vi "Set 2D Ramp Rates_manual_ramp_brasse.vi"(0 "Y-Axis Communications Config":T1={"GPIB address"=22, "GPIB bus"=0, "connection ID"=refnum, "IP"="192.168.2.200", "Active Comm Interface"=0, "Serial Port"="", "Programmer Type"=0} {"Programmer Type" items=["Model 430", "Model 420"]; "Active Comm Interface" items=["TCP/IP (Model 430 Only)", "RS232", "IEEE488"]}, 1 "Y-Axis Field (kG)":dbl format="%.3f", 3 "Next Y-Axis Field (kG)":dbl format="%.3f", 4 "Z-Axis Communications Config":T1={"GPIB address"=22, "GPIB bus"=0, "connection ID"=refnum, "IP"="192.168.2.200", "Active Comm Interface"=0, "Serial Port"="", "Programmer Type"=0} {"Programmer Type" items=["Model 430", "Model 420"]; "Active Comm Interface" items=["TCP/IP (Model 430 Only)", "RS232", "IEEE488"]}, 5 "Z-Axis Field (kG)":dbl format="%.3f", 6 "User defined Ramp Rate (T/min)":bool, 7 "Next Z-Axis Field (kG)":dbl format="%.3f", 8 "Max Ramp Rate - Y Axis (A/s)":dbl format="%.3f", 9 "Max Ramp Rate - Z Axis (A/s)":dbl format="%.3f", 10 "User defined Ramp Rate - Z Axis (kG/s)":dbl format="%.3f", 11 "error in":T2, 12 "User defined Ramp Rate Y-Axis (kG/s)":dbl format="%.3f") -> (15 "Y-Axis Ramp Rate (T/min)":dbl format="%.3f", 17 "Z-Axis Ramp Rate (T/min)":dbl format="%.3f", 18 "error out":T2)   [LabVIEW 2009]
panel:
  in  "Z-Axis Communications Config 4":T1={"GPIB address"=22, "GPIB bus"=0, "connection ID"=refnum, "IP"="192.168.2.200", "Active Comm Interface"=0, "Serial Port"="", "Programmer Type"=0} {"Programmer Type" items=["Model 430", "Model 420"]; "Active Comm Interface" items=["TCP/IP (Model 430 Only)", "RS232", "IEEE488"]}
  in  "Z-Axis Communications Config 3":T1={"GPIB address"=22, "GPIB bus"=0, "connection ID"=refnum, "IP"="192.168.2.200", "Active Comm Interface"=0, "Serial Port"="", "Programmer Type"=0} {"Programmer Type" items=["Model 430", "Model 420"]; "Active Comm Interface" items=["TCP/IP (Model 430 Only)", "RS232", "IEEE488"]}
  in  "Z-Axis Communications Config 2":T1={"GPIB address"=22, "GPIB bus"=0, "connection ID"=refnum, "IP"="192.168.2.200", "Active Comm Interface"=0, "Serial Port"="", "Programmer Type"=0} {"Programmer Type" items=["Model 430", "Model 420"]; "Active Comm Interface" items=["TCP/IP (Model 430 Only)", "RS232", "IEEE488"]}
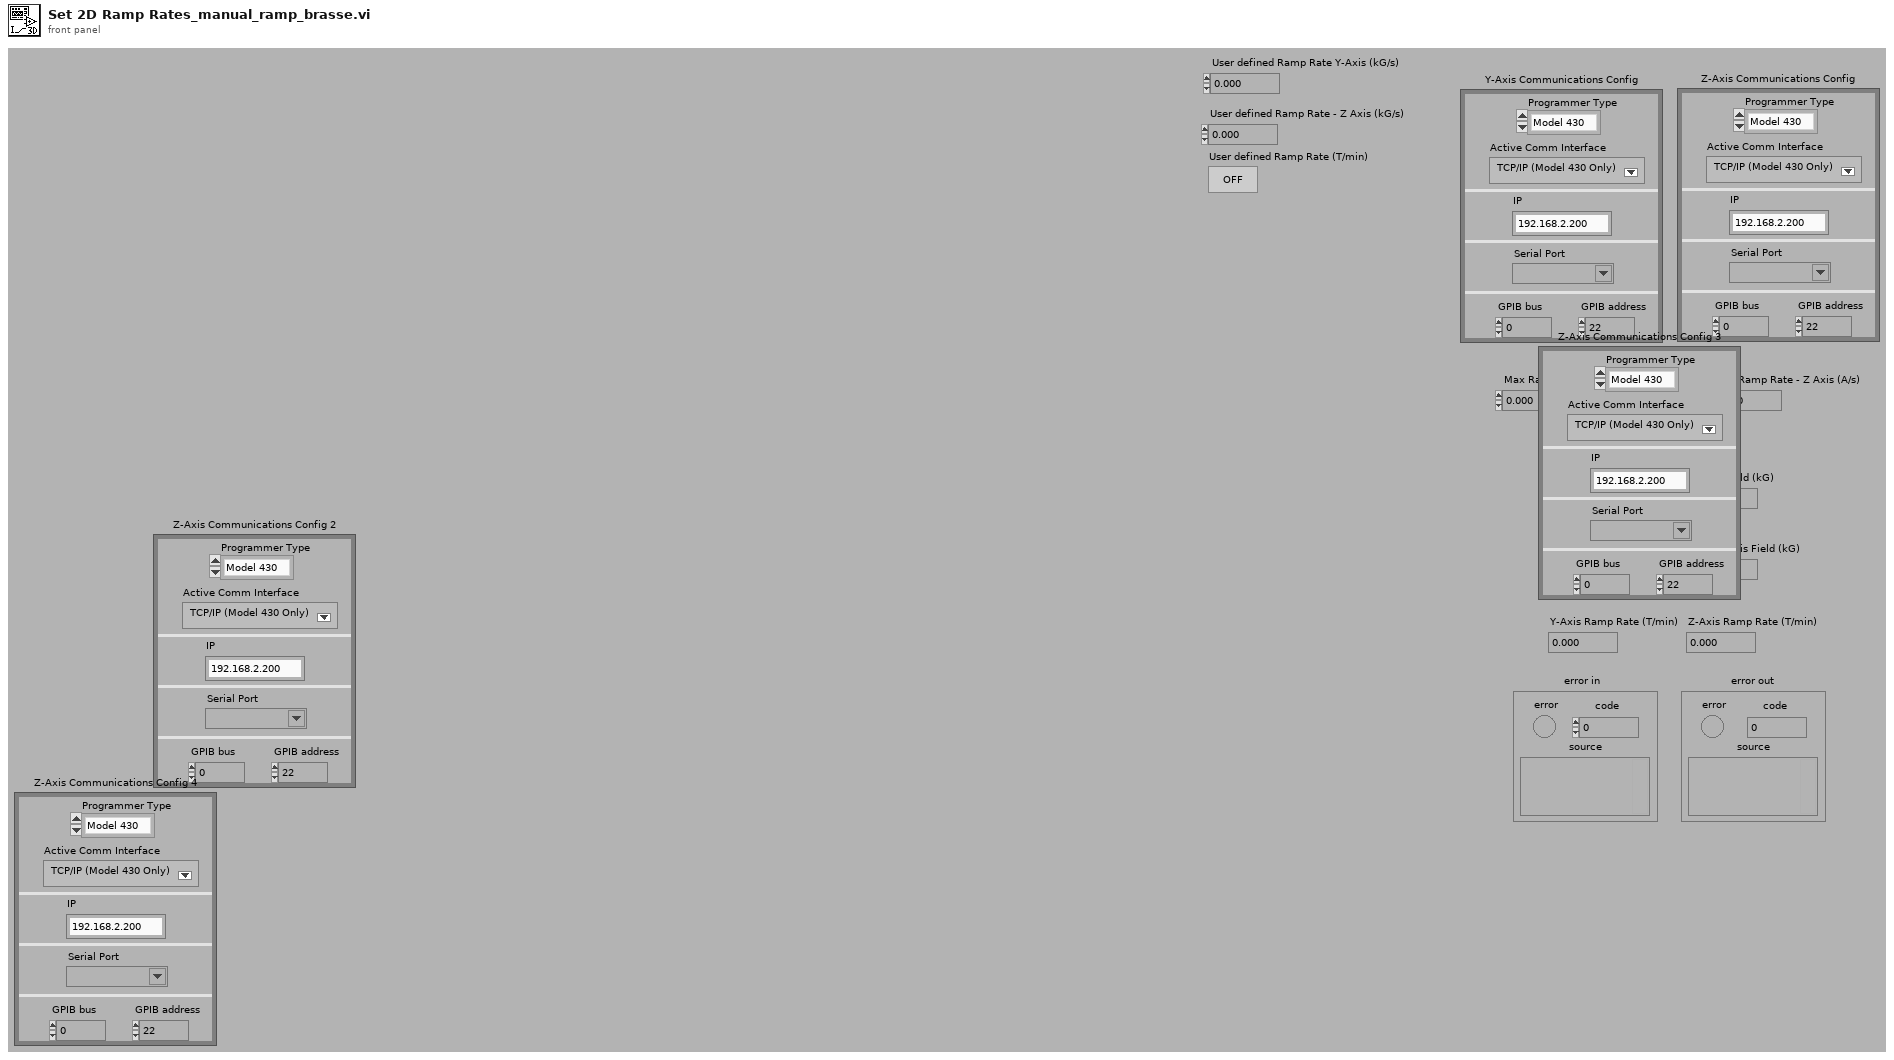
[diagram p1: front panel]
types:
  T1 = cluster{"GPIB address":i16, "GPIB bus":i16, "connection ID":refnum<k5>, "IP":string, "Active Comm Interface":u16, "Serial Port":refnum<visa-resource-name>, "Programmer Type":u16}
  T2 = cluster{"error":bool, "code":i32, "source":string}
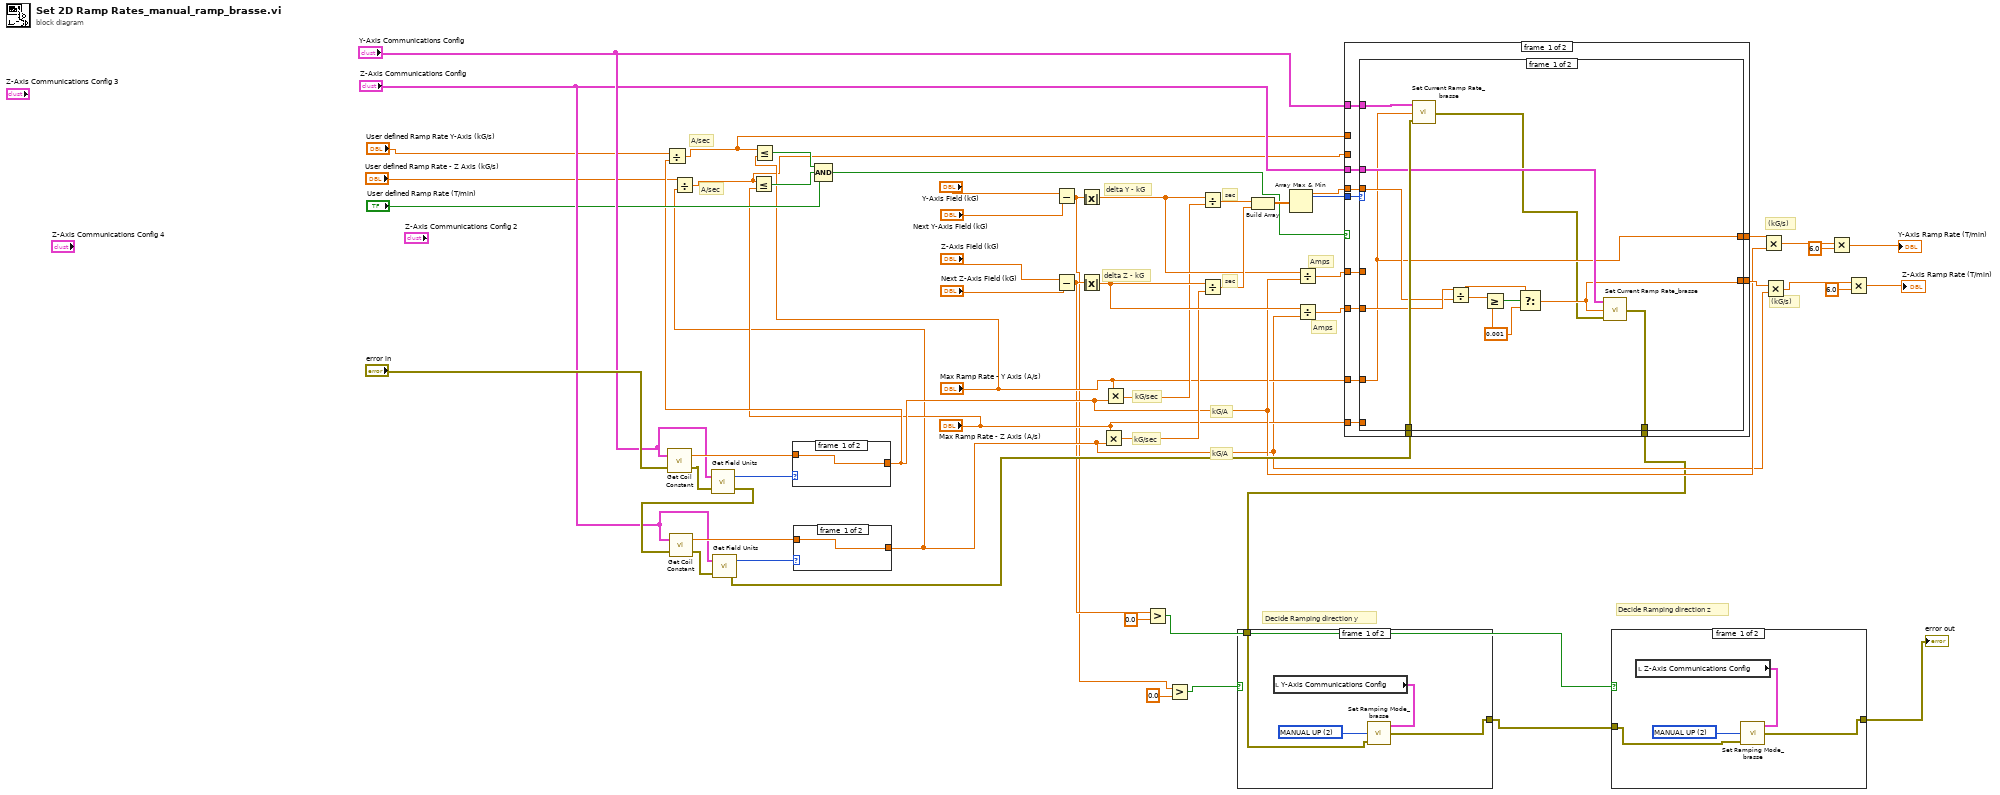
[diagram p0: block diagram]
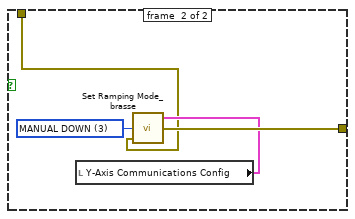
[diagram p2: hidden frame]
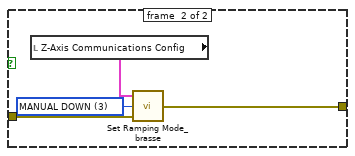
[diagram p3: hidden frame]
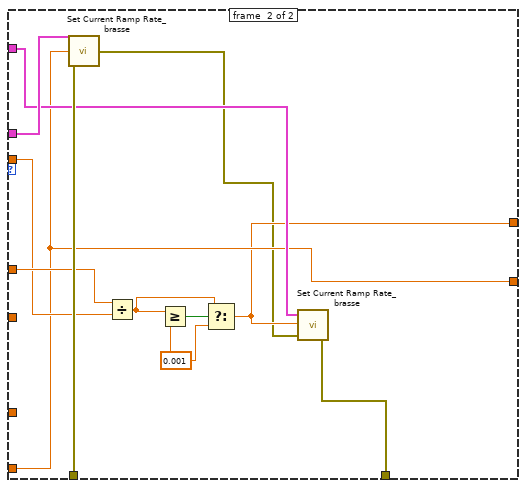
[diagram p4: hidden frame]
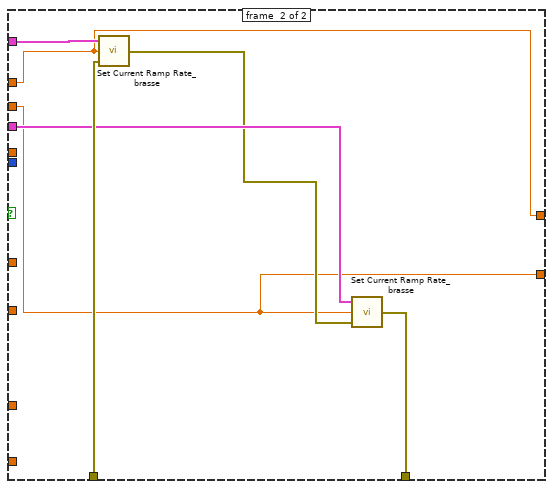
[diagram p5: hidden frame]
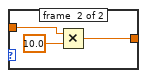
[diagram p6: hidden frame]
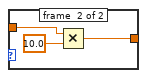
[diagram p7: hidden frame]
diagram:
  # "Decide Ramping direction y"
  # "Decide Ramping direction z"
  # "(kG/s)"
  # "(kG/s)"
  # "A/sec"
  # "A/sec"
  # "Amps"
  # "Amps"
  # "kG/A"
  # "kG/A"
  # "kG/sec"
  # "kG/sec"
  # "delta Z - kG"
  # "delta Y - kG"
  # "sec"
  # "sec"
  n1 = call <userlib>:"Get Coil Constant.vi"("error in"="error in", "Communications Config"="Y-Axis Communications Config") -> ("error out"=w38:T2, "Coil Constant"=w39:dbl)
  n2 = call <userlib>:"Get Field Units.vi"("error in"=w38, "Communications Config"="Y-Axis Communications Config") -> ("error out"=w34:T2, "Field Units"=w40:enum16{"kg", "t"})
  n3 = call <userlib>:"Get Coil Constant.vi"("error in"=w34, "Communications Config"="Z-Axis Communications Config") -> ("error out"=w35:T2, "Coil Constant"=w36:dbl)
  n4 = call <userlib>:"Get Field Units.vi"("error in"=w35, "Communications Config"="Z-Axis Communications Config") -> ("error out"=w33:T2, "Field Units"=w37:enum16{"kg", "t"})
  n5 = case shown="\"t\"" w40 {
    tunnel: w39 -> [w56 w58]
    tunnel: [w56 w57] -> w21
    frame #0 {
    }
    frame #1 {
      n6 = Multiply(x=w58, y=10.0) -> (x*y=w57:dbl)
    }
  }
  n7 = Divide(x="User defined Ramp Rate Y-Axis (kG/s)", y=w21) -> (x/y=w22:dbl)
  n8 = Less Or Equal?(x=w22, y="Max Ramp Rate - Y Axis (A/s)") -> (x <= y?=w27:bool)
  n9 = case shown="\"t\"" w37 {
    tunnel: w36 -> [w60 w62]
    tunnel: [w60 w61] -> w17
    frame #0 {
    }
    frame #1 {
      n10 = Multiply(x=w62, y=10.0) -> (x*y=w61:dbl)
    }
  }
  n11 = Divide(x="User defined Ramp Rate - Z Axis (kG/s)", y=w17) -> (x/y=w16:dbl)
  n12 = Less Or Equal?(x=w16, y="Max Ramp Rate - Z Axis (A/s)") -> (x <= y?=w26:bool)
  n13 = Compound Arithmetic op=AND(w27, w26, "User defined Ramp Rate (T/min)") -> (w24:bool)
  n14 = Subtract(x="Y-Axis Field (kG)", y="Next Y-Axis Field (kG)") -> (x-y=w2:dbl)
  n15 = Subtract(x="Z-Axis Field (kG)", y="Next Z-Axis Field (kG)") -> (x-y=w9:dbl)
  n16 = Absolute Value(x=w2) -> (abs(x)=w47:dbl)
  n17 = Absolute Value(x=w9) -> (abs(x)=w46:dbl)
  n18 = Multiply(x="Max Ramp Rate - Z Axis (A/s)", y=w17) -> (x*y=w29:dbl)
  n19 = Multiply(x="Max Ramp Rate - Y Axis (A/s)", y=w21) -> (x*y=w28:dbl)
  n20 = Greater?(x=w9, y=0.0) -> (0:w8:bool)
  n21 = Greater?(x=w2, y=0.0) -> (0:w1:bool)
  n22 = Divide(x=w47, y=w28) -> (x/y=w55:dbl)
  n23 = Divide(x=w46, y=w29) -> (x/y=w54:dbl)
  n24 = Build Array(w55, w54) -> (w48:dbl[])
  n25 = Array Max & Min(array=w48) -> (max value=w45:dbl, max index (indices)=w49:i32)  [unwired: 2 out]
  n26 = Divide(x=w47, y=w21) -> (x/y=w44:dbl)
  n27 = Divide(x=w46, y=w17) -> (x/y=w43:dbl)
  n28 = case shown="False" w24 {
    tunnel: w49 -> [w75 _]
    tunnel: w45 -> [w74 _]
    tunnel: w44 -> [w73 _]
    tunnel: w43 -> [w72 _]
    tunnel: [w71 w101] -> w42
    tunnel: [w70 w100] -> w41
    tunnel: w33 -> [w69 w106]
    tunnel: "Max Ramp Rate - Y Axis (A/s)" -> [w68 _]
    tunnel: "Max Ramp Rate - Z Axis (A/s)" -> [w67 _]
    tunnel: [w66 w105] -> w5
    tunnel: "Y-Axis Communications Config" -> [w65 w104]
    tunnel: "Z-Axis Communications Config" -> [w64 w103]
    tunnel: w22 -> [_ w101]
    tunnel: w16 -> [_ w100]
    frame #0 {
      n29 = case shown="1" w75 {
        tunnel: w69 -> [w86 w98]
        tunnel: w74 -> [w84 w96]
        tunnel: w73 -> [_ w97]
        tunnel: w65 -> [w87 w95]
        tunnel: w72 -> [w85 _]
        tunnel: w64 -> [w83 w99]
        tunnel: [w82 w94] -> w66
        tunnel: [w81 w89] -> w71
        tunnel: [w77 w93] -> w70
        tunnel: w68 -> [w81 _]
        tunnel: w67 -> [_ w93]
        frame #0 {
          w80 = 0.001 ("f")
          n30 = call "Set Current Ramp Rate_brasse.vi"("Communications Config"=w87, "Ramp Rate (A/sec)"=w81, "error in"=w86) -> ("error out"=w76:T2)  [unwired: 2 in]
          n31 = Divide(x=w85, y=w84) -> (x/y=w78:dbl)
          n32 = Greater Or Equal?(x=w78, y=w80) -> (x >= y?=w79:bool)
          n33 = Select(t=w78, s=w79, f=w80) -> (s? t:f=w77:dbl)
          n34 = call "Set Current Ramp Rate_brasse.vi"("Communications Config"=w83, "Ramp Rate (A/sec)"=w77, "error in"=w76) -> ("error out"=w82:T2)  [unwired: 2 in]
        }
        frame #1 {
          w92 = 0.001 ("f")
          n35 = call "Set Current Ramp Rate_brasse.vi"("Communications Config"=w99, "Ramp Rate (A/sec)"=w93, "error in"=w98) -> ("error out"=w88:T2)  [unwired: 2 in]
          n36 = Divide(x=w97, y=w96) -> (x/y=w90:dbl)
          n37 = Greater Or Equal?(x=w90, y=w92) -> (x >= y?=w91:bool)
          n38 = Select(t=w90, s=w91, f=w92) -> (s? t:f=w89:dbl)
          n39 = call "Set Current Ramp Rate_brasse.vi"("Communications Config"=w95, "Ramp Rate (A/sec)"=w89, "error in"=w88) -> ("error out"=w94:T2)  [unwired: 2 in]
        }
      }
    }
    frame #1 {
      n40 = call "Set Current Ramp Rate_brasse.vi"("Communications Config"=w104, "Ramp Rate (A/sec)"=w101, "error in"=w106) -> ("error out"=w102:T2)  [unwired: 2 in]
      n41 = call "Set Current Ramp Rate_brasse.vi"("Communications Config"=w103, "Ramp Rate (A/sec)"=w100, "error in"=w102) -> ("error out"=w105:T2)  [unwired: 2 in]
    }
  }
  n42 = case shown="True" w1 {
    tunnel: [w109 w114] -> w4
    tunnel: w5 -> [w107 w111]
    frame #0 {
      w110 = u16 2 items=["RAMP", "PAUSE", "MANUAL UP", "MANUAL DOWN", "ZERO"] ("Ramping Mode")
      n43 = local read "Y-Axis Communications Config"() -> (w108:T1)
      n44 = call "Set Ramping Mode_brasse.vi"("error in"=w107, "Ramping Mode"=w110, "Communications Config"=w108) -> ("error out"=w109:T2)
    }
    frame #1 {
      w113 = u16 3 items=["RAMP", "PAUSE", "MANUAL UP", "MANUAL DOWN", "ZERO"] ("Ramping Mode")
      n45 = local read "Y-Axis Communications Config"() -> (w112:T1)
      n46 = call "Set Ramping Mode_brasse.vi"("error in"=w111, "Ramping Mode"=w113, "Communications Config"=w112) -> ("error out"=w114:T2)
    }
  }
  n47 = case shown="False" w8 {
    tunnel: [w116 w121] -> w6
    tunnel: w4 -> [w117 w120]
    frame #0 {
      w118 = u16 2 items=["RAMP", "PAUSE", "MANUAL UP", "MANUAL DOWN", "ZERO"] ("Ramping Mode")
      n48 = local read "Z-Axis Communications Config"() -> (w115:T1)
      n49 = call "Set Ramping Mode_brasse.vi"("error in"=w117, "Ramping Mode"=w118, "Communications Config"=w115) -> ("error out"=w116:T2)
    }
    frame #1 {
      w119 = u16 3 items=["RAMP", "PAUSE", "MANUAL UP", "MANUAL DOWN", "ZERO"] ("Ramping Mode")
      n50 = local read "Z-Axis Communications Config"() -> (w122:T1)
      n51 = call "Set Ramping Mode_brasse.vi"("error in"=w120, "Ramping Mode"=w119, "Communications Config"=w122) -> ("error out"=w121:T2)
    }
  }
  "error out" <- w6
  n52 = Multiply(x=w42, y=w21) -> (x*y=w12:dbl)
  n53 = Multiply(x=w41, y=w17) -> (x*y=w15:dbl)
  n54 = Multiply(x=w12, y=6.0) -> (x*y=→"Y-Axis Ramp Rate (T/min)":dbl)
  n55 = Multiply(x=w15, y=6.0) -> (x*y=→"Z-Axis Ramp Rate (T/min)":dbl)
